vi "Treatment of NaN and Inf.vi"(7 "enable LabVIEW extensions?":bool, 11 "Numeric Text":string) -> (3 "<JSON>":string)   [LabVIEW 2019, in "JSONtext.lvlib"]
uses:
  JSONtext.lvlib
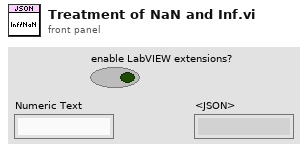
[diagram p1: front panel]
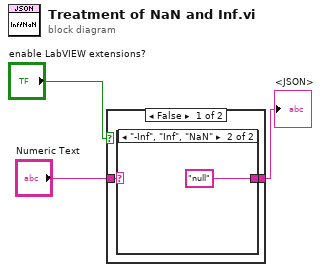
[diagram p0: block diagram]
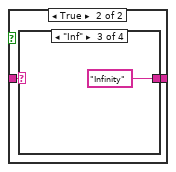
[diagram p3: hidden frame]
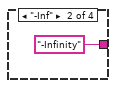
[diagram p5: hidden frame]
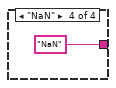
[diagram p6: hidden frame]
diagram:
  n1 = case shown="False" "enable LabVIEW extensions?" {
    tunnel: "Numeric Text" -> [w5 w9]
    tunnel: [w4 w8] -> w2
    frame False {
      n2 = case shown="\"-Inf\", \"Inf\", \"NaN\"" w5 {
        selector: w5 -> [w6 _]
        tunnel: [w6 "null"] -> w4
        frame Default {
        }
        frame "-Inf", "Inf", "NaN" {
        }
      }
    }
    frame True {
      n3 = case shown="\"Inf\"" w9 {
        selector: w9 -> [w10 _ _ _]
        tunnel: [w10 "-Infinity" "Infinity" "NaN"] -> w8
        frame Default {
        }
        frame "-Inf" {
        }
        frame "Inf" {
        }
        frame "NaN" {
        }
      }
    }
  }
  "<JSON>" <- w2
